vi "Start Disconnect.vi"(8 "error in (no error)":errorcluster, 11 "TCP Comm":T1) -> (0 "error out":errorcluster)   [LabVIEW 2020, in "TCP Comms.lvlib"]
uses:
  TCP Comms.lvlib
  TCP Comm.ctl
  Ref Data.ctl
  State.ctl
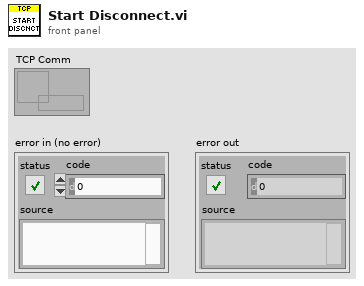
[diagram p1: front panel]
types:
  T1 = typedef "TCP Comms.lvlib/TCP Comm.ctl" = refnum<data-value>
  T2 = typedef "TCP Comms.lvlib/State.ctl" = enum16{"Idle", "Starting", "Connecting", "Connected", "Disconnecting", "Stopped"}
  T3 = typedef "TCP Comms.lvlib/Ref Data.ctl" = cluster{"TCP":refnum<k5>, "State":T2, "Server":bool, "Host":string, "Port":u16, "Listener":refnum<k5>, "Start":bool, "Disconnect":bool, "TCP Valid":bool, "TLS Enabled":bool, "Immutable TLS":refnum<k36>, "Certificate DN":string}
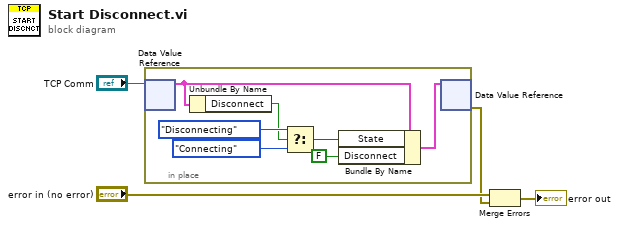
[diagram p0: block diagram]
diagram:
  n1 = in-place {
    n2 = in-place-dvr #1("TCP Comm") -> (w6:T3)  [unwired: 1 out]
    n3 = Unbundle By Name(w6) -> ("Disconnect"=w5:bool)
    n4 = Select(t=State."Disconnecting" ("State"), s=w5, f=State."Connecting" ("State")) -> (s? t:f=w7:T2)
    n5 = Bundle By Name(cluster=w6, "State"=w7, "Disconnect"=FALSE) -> (w11:T3)
    n6 = in-place-dvr #1(w11) -> (w2:errorcluster)  [unwired: 1 out]
  }
  n7 = Merge Errors("error in (no error)", w2) -> (→"error out":errorcluster)
